vi "setPhaseBlazingTable.vi"(2 "-¹..¹ range control":enum16{"wrap round", "cast to range"}(ring)=enum."cast to range", 3 "Anchor Points":cluster{"X":dbl, "Y":dbl}[](array[cluster])=[{"X"=-3.141592653589793, "Y"=0.0}, {"X"=3.141592653589793, "Y"=1.0}, {"X"=-1.4364705882352942, "Y"=0.07537688442211056}, {"X"=2.737058823529411, "Y"=0.2914572864321608}], 4 "#elements (default 256)":i32=256) -> (0 "blazing graph":cluster{dbl, dbl}[](graph)=[{-3.141592653589793, 0.0}, {-2.938909256584, 0.03548443703005898}, {-2.736225859578207, 0.06868797880673808}, {-2.533542462572414, 0.09732973007665743}, {-2.330859065566621, 0.11912879558643716}, {-2.1281756685608277, 0.1318042800826974}, {-1.9254922715550344, 0.13307528831205828}, {-1.7228088745492414, 0.12066092502113993}, {-1.5201254775434483, 0.09228029495656248}, {-1.317442080537655, 0.045850300167624036}, {-1.114758683531862, 0.0}, {-0.9120752865260688, 0.0}, {-0.7093918895202758, 0.0}, {-0.5067084925144827, 0.0}, {-0.3040250955086896, 0.0}, {-0.10134169850289654, 0.0}, {0.10134169850289654, 0.0}, {0.30402509550868917, 0.0}, {0.5067084925144831, 0.0}, {0.7093918895202758, 0.0}, {0.9120752865260693, 0.0}, {1.1147586835318615, 0.0}, {1.3174420805376554, 0.0}, {1.5201254775434485, 0.0}, {1.7228088745492416, 0.0}, {1.9254922715550338, 0.0}, {2.1281756685608277, 0.0}, {2.330859065566621, 0.0}, {2.533542462572414, 0.0}, {2.736225859578207, 0.29014782740336237}, {2.938909256584, 0.6314200278304355}, {3.141592653589793, 1.0}], 1 "blazing table":dbl[](array[numeric])=[0.0, 0.03548443703005898, 0.06868797880673808, 0.09732973007665743, 0.11912879558643716, 0.1318042800826974, 0.13307528831205828, 0.12066092502113993, 0.09228029495656248, 0.045850300167624036, 0.0, 0.0, 0.0, 0.0, 0.0, 0.0, 0.0, 0.0, 0.0, 0.0, 0.0, 0.0, 0.0, 0.0, 0.0, 0.0, 0.0, 0.0, 0.0, 0.29014782740336237, 0.6314200278304355, 1.0])   [LabVIEW 2020]
uses:
  <vilib>/Analysis/NI_AALPro.lvlib
panel:
  # "This should have range 0 to 1, with -pi->pi mapped onto the range if its indices for X"
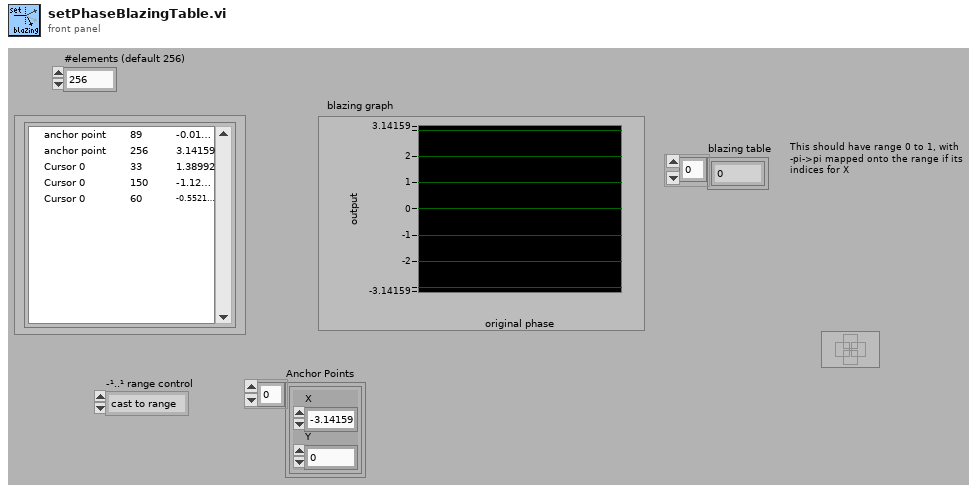
[diagram p1: front panel]
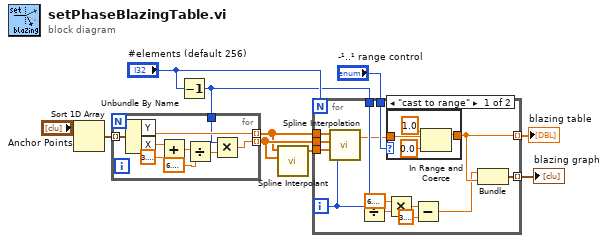
[diagram p0: block diagram]
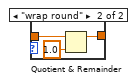
[diagram p2: hidden frame]
diagram:
  n1 = Sort 1D Array(array="Anchor Points") -> (sorted array=w7:cluster{"X":dbl, "Y":dbl}[])
  n2 = Decrement(x="#elements (default 256)") -> (x-1=w4:i32)
  n3 = for {
    tunnel: w7 -> [w19] mode=indexing
    tunnel: [w18] -> w9 mode=indexing
    tunnel: [w12] -> w10 mode=indexing
    tunnel: w4 -> [w11]
    n4 = Unbundle By Name(w19) -> ("Y"=w18:dbl, "X"=w17:dbl)
    n5 = Add(x=w17, y=3.141592653589793) -> (x+y=w15:dbl)
    n6 = Divide(x=w15, y=6.283185307179586) -> (x/y=w13:dbl)
    n7 = Multiply(x=w11, y=w13) -> (x*y=w12:dbl)
  }
  n8 = call <vilib>:"Spline Interpolant.vi"("X"=w10, "Y"=w9) -> ("Interpolant"=w8:dbl[])  [unwired: 2 in, 1 out]
  n9 = for {
    N: "#elements (default 256)" -> [_]
    tunnel: w8 -> [w33]
    tunnel: w9 -> [w32]
    tunnel: w10 -> [w31]
    tunnel: w4 -> [w29]
    tunnel: "-¹..¹ range control" -> [w24]
    tunnel: [w21] -> w2 mode=indexing
    tunnel: [w22] -> w1 mode=indexing
    i -> [w30]
    n10 = call <vilib>:"Spline Interpolation.vi"("x value"=w30, "Interpolant"=w33, "X"=w31, "Y"=w32) -> ("interpolation value"=w23:dbl)  [unwired: 1 out]
    n11 = Divide(x=w30, y=w29) -> (x/y=w28:dbl)
    n12 = Multiply(x=6.283185307179586, y=w28) -> (x*y=w26:dbl)
    n13 = case shown="\"cast to range\"" w24 {
      tunnel: [w34 w38] -> w21
      tunnel: w23 -> [w37 w40]
      frame "cast to range" {
        n14 = In Range and Coerce(upper limit=1.0 ("x"), x=w37, lower limit=0.0 ("x")) -> (coerced(x)=w34:dbl)  [unwired: 1 out]
      }
      frame "wrap round" {
        n15 = Quotient & Remainder(x=w40, y=1.0) -> (x-y*floor(x/y)=w38:dbl)  [unwired: 1 out]
      }
    }
    n16 = Subtract(x=w26, y=3.141592653589793) -> (x-y=w20:dbl)
    n17 = Bundle(w20, "x"=w21) -> (w22:cluster{dbl, "x":dbl})  [unwired: 1 out]
  }
  "blazing graph" <- w1
  "blazing table" <- w2
